vi "Create Sections and Channels.vi"(8 "error in (no error)":errorcluster, 10 "Configuration":T1={"Name"="", "Description"="", "Diagnostics Basic Configuraiton"={"Database File"=path "", "CAN Interface"=enum."CAN0", "Baud Rate"=0, "Diagnostic Protocol"=enum."GMLAN", "Transport Protocol"=enum."ISO TP - Normal Mode", "Transmit ID"=0, "Receive ID"=0, "Transmit Extension"=0, "Receive Extension"=0, "Receive UUDT ID"=0, "Enable Stream"=TRUE, "VW TP Channel ID"=0}, "DIDs"={"Description"="", "DIDPID Array"=[]}, "Input PIDs"={"Description"="", "DIDPID Array"=[]}, "Output PIDs"={"Description"="", "DIDPID Array"=[]}, "DPIDs"={"Description"="", "DPIDs"=[]}, "DTC"={"Description"="", "DTC descriptor"={"DTC Byte Length"=2, "Status Byte Length"=1, "Add Data Byte Length"=1, "Byte Order"=enum."Motorola"}}, "NI 986x Support"={"Enable 986x"=FALSE, "RIO Device"=0, "Bitfile"=path ""}, "Commands"={"Description"=""}, "Status"={"Description"=""}} {"Diagnostics Basic Configuraiton"."VW TP Channel ID" format="%.0x"; "Diagnostics Basic Configuraiton"."Receive UUDT ID" format="%.0x"; "Diagnostics Basic Configuraiton"."Receive Extension" format="%.0x"; "Diagnostics Basic Configuraiton"."Transmit Extension" format="%.0x"; "Diagnostics Basic Configuraiton"."Receive ID" format="%.0x"; "Diagnostics Basic Configuraiton"."Transmit ID" format="%.0x"; "DIDs"."DIDPID Array"."Signals"."Byte Order" items=["Little Endian", "Big Endian"]; "DIDs"."DIDPID Array"."Signals"."Data Type" items=["Signed", "Unsigned", "IEEE Float"]; "Input PIDs"."DIDPID Array"."Signals"."Byte Order" items=["Little Endian", "Big Endian"]; "Input PIDs"."DIDPID Array"."Signals"."Data Type" items=["Signed", "Unsigned", "IEEE Float"]; "Output PIDs"."DIDPID Array"."Signals"."Byte Order" items=["Little Endian", "Big Endian"]; "Output PIDs"."DIDPID Array"."Signals"."Data Type" items=["Signed", "Unsigned", "IEEE Float"]}, 11 "Device Item Ref in":T18 format="%.0x") -> (0 "error out":errorcluster, 3 "Device Item Ref out":T18 format="%.0x")   [LabVIEW 2013, in "Diagnostics Addon Shared.lvlib"]
uses:
  Diagnostics Addon Shared.lvlib
  <vilib>/NI Veristand/Custom Device API/Custom Device Item Ref.ctl
  Exported Configuration.ctl
  CAN Configuration.ctl
  CAN Interface.ctl
  Diagnostic Protocols.ctl
  Transport Protocols.ctl
  Exported DIDPIDs Cluster.ctl
  DIDPID Parameters.ctl
  DIDPID Signal Parameters.ctl
  Exported DPIDs Cluster.ctl
  Exported DPID Parameters.ctl
  DPID Parameters.ctl
  DPID Periodic Rate.ctl
  Exported DTC Cluster.ctl
  <vilib>/Automotive Diagnostic Command Set/Diagnostic Protocols.llb/DTC Descriptor.ctl
  Exported 986x Support.ctl
  Exported Command Cluster.ctl
  Exported Status Cluster.ctl
  <vilib>/NI Veristand/Custom Device API/Custom Device Channel.ctl
  <vilib>/NI Veristand/Custom Device API/Custom Device Channel Type.ctl
  FG Action.ctl
  GUID Lookup.vi
  <vilib>/NI Veristand/Custom Device API/NI VeriStand - Set Item Property.vi
  <vilib>/NI Veristand/Custom Device API/Set Item Property (Variant).vi
  <vilib>/NI Veristand/Custom Device API/Custom Device API.lvlib
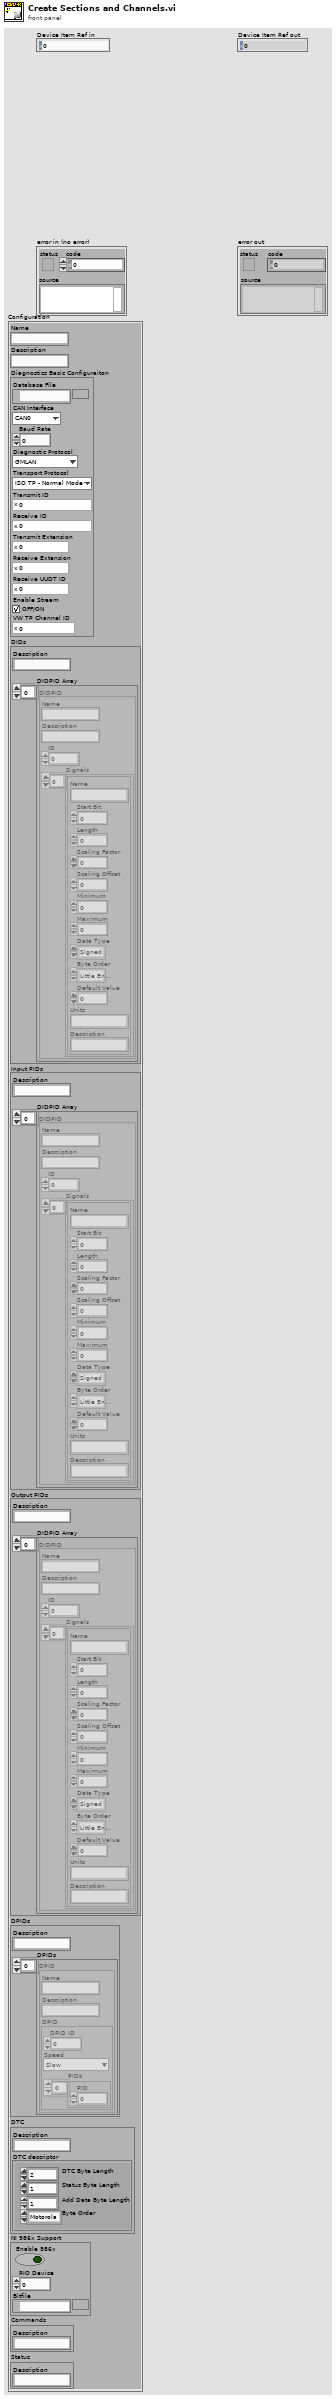
[diagram p1: front panel]
types:
  T1 = typedef "Diagnostics Addon Shared.lvlib/Exported Configuration.ctl" = cluster{"Name":string, "Description":string, "Diagnostics Basic Configuraiton":T2, "DIDs":T6, "Input PIDs":T6, "Output PIDs":T6, "DPIDs":T9, "DTC":T13, "NI 986x Support":T15, "Commands":T16, "Status":T17}
  T2 = typedef "Diagnostics Addon Shared.lvlib/CAN Configuration.ctl" = cluster{"Database File":path, "CAN Interface":T3, "Baud Rate":u32, "Diagnostic Protocol":T4, "Transport Protocol":T5, "Transmit ID":u32, "Receive ID":u32, "Transmit Extension":u8, "Receive Extension":u8, "Receive UUDT ID":u32, "Enable Stream":bool, "VW TP Channel ID":u32}
  T3 = typedef "Diagnostics Addon Shared.lvlib/CAN Interface.ctl" = enum16{"CAN0", "CAN1", "CAN2", "CAN3", "CAN4", "CAN5", "CAN6", "CAN7", "CAN8", "CAN9", "CAN10", "CAN11", "CAN12", "CAN13", "CAN14", "CAN15", "CAN16", "CAN17", "CAN18", "CAN19", "CAN20", "CAN21", "CAN22", "CAN23", "CAN24", "CAN25", "CAN26", "CAN27", "CAN28", "CAN29", "CAN30", "CAN31", "CAN32", "CAN33", "CAN34", "CAN35", "CAN36", "CAN37", "CAN38", "CAN39", "CAN40", "CAN41", "CAN42", "CAN43", "CAN44", "CAN45", "CAN46", "CAN47", "CAN48", "CAN49", "CAN50", "CAN51", "CAN52", "CAN53", "CAN54", "CAN55", "CAN56", "CAN57", "CAN58", "CAN59", "CAN60", "CAN61", "CAN62", "CAN63", "CAN 256 (Virtual)", "CAN 257 (Virtual)"}
  T4 = typedef "Diagnostics Addon Shared.lvlib/Diagnostic Protocols.ctl" = enum16{"GMLAN", "KWP-2000", "UDS"}
  T5 = typedef "Diagnostics Addon Shared.lvlib/Transport Protocols.ctl" = enum16{"ISO TP - Normal Mode", "ISO TP - Mixed Mode", "VW TP 2.0", "Diagnostics on IP"}
  T6 = typedef "Diagnostics Addon Shared.lvlib/Exported DIDPIDs Cluster.ctl" = cluster{"Description":string, "DIDPID Array":T7[]}
  T7 = typedef "Diagnostics Addon Shared.lvlib/DIDPID Parameters.ctl" = cluster{"Name":string, "Description":string, "ID":u16, "Signals":T8[]}
  T8 = typedef "Diagnostics Addon Shared.lvlib/DIDPID Signal Parameters.ctl" = cluster{"Name":string, "Start Bit":u8, "Length":u8, "Scaling Factor":dbl, "Scaling Offset":dbl, "Minimum":dbl, "Maximum":dbl, "Data Type":u32, "Byte Order":u32, "Default Value":dbl, "Units":string, "Description":string}
  T9 = typedef "Diagnostics Addon Shared.lvlib/Exported DPIDs Cluster.ctl" = cluster{"Description":string, "DPIDs":T10[]}
  T10 = typedef "Diagnostics Addon Shared.lvlib/Exported DPID Parameters.ctl" = cluster{"Name":string, "Description":string, "DPID":T11}
  T11 = typedef "Diagnostics Addon Shared.lvlib/DPID Parameters.ctl" = cluster{"DPID ID":u8, "Speed":T12, "PIDs":u16[]}
  T12 = typedef "Diagnostics Addon Shared.lvlib/DPID Periodic Rate.ctl" = enum16{"Slow", "Medium", "Fast"}
  T13 = typedef "Diagnostics Addon Shared.lvlib/Exported DTC Cluster.ctl" = cluster{"Description":string, "DTC descriptor":T14}
  T14 = typedef "DTC Descriptor.ctl" = cluster{"DTC Byte Length":i32, "Status Byte Length":i32, "Add Data Byte Length":i32, "Byte Order":enum16{"Motorola", "Intel"}}
  T15 = typedef "Diagnostics Addon Shared.lvlib/Exported 986x Support.ctl" = cluster{"Enable 986x":bool, "RIO Device":u16, "Bitfile":path}
  T16 = typedef "Diagnostics Addon Shared.lvlib/Exported Command Cluster.ctl" = cluster{"Description":string}
  T17 = typedef "Diagnostics Addon Shared.lvlib/Exported Status Cluster.ctl" = cluster{"Description":string}
  T18 = typedef "Custom Device API.lvlib/Custom Device Item Ref.ctl" = u64
  T19 = typedef "Diagnostics Addon Shared.lvlib/FG Action.ctl" = enum16{"Get", "Set"}
  T20 = typedef "Custom Device API.lvlib/Custom Device Channel.ctl" = cluster{"Type":T21, "Units":string, "Default Value":dbl, "Faultable":bool, "Scalable":bool}
  T21 = typedef "Custom Device API.lvlib/Custom Device Channel Type.ctl" = enum16{"Input", "Output"}
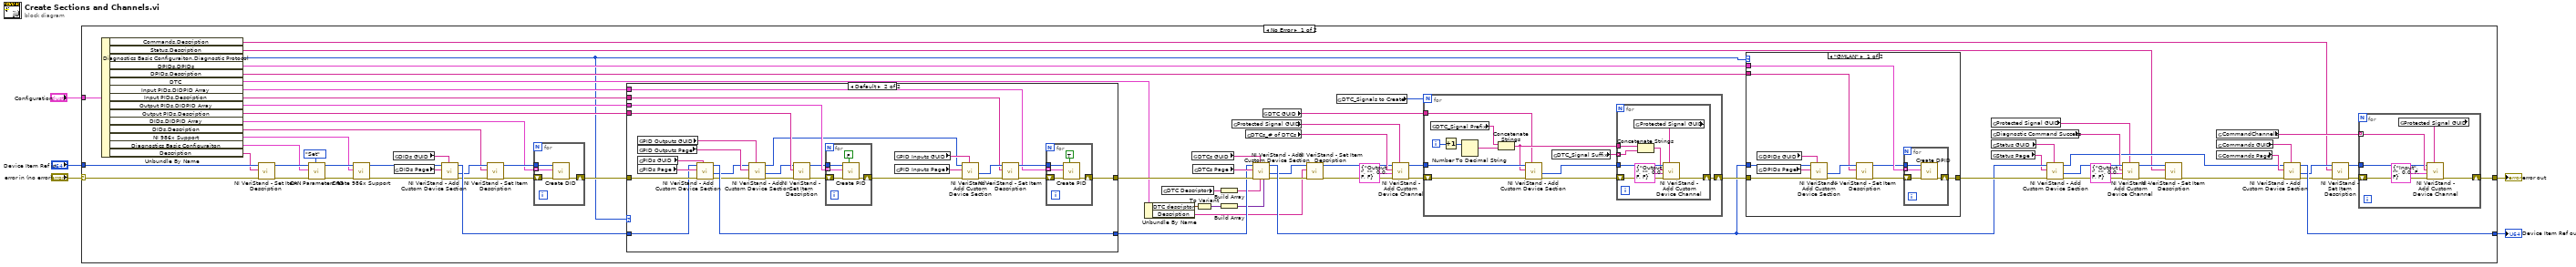
[diagram p0: block diagram]
diagram:
  n1 = case shown="No Error" "error in (no error)" {
    selector: "error in (no error)" -> [w44 w168]
    tunnel: [w54 w168] -> w4
    tunnel: "Device Item Ref in" -> [w48 w167]
    tunnel: [w52 w167] -> w2
    tunnel: "Configuration" -> [w47 _]
    frame No Error {
      n2 = Unbundle By Name(w47) -> ("Commands.Description"=w12:string, "Status.Description"=w13:string, "Diagnostics Basic Configuraiton.Diagnostic Protocol"=w6:T4, "DPIDs.DPIDs"=w22:T10[], "DPIDs.Description"=w21:string, "DTC"=w29:T13, "Input PIDs.DIDPID Array"=w32:T7[], "Input PIDs.Description"=w33:string, "Output PIDs.DIDPID Array"=w31:T7[], "Output PIDs.Description"=w34:string, "DIDs.DIDPID Array"=w35:T7[], "DIDs.Description"=w36:string, "NI 986x Support"=w7:T15, "Diagnostics Basic Configuraiton"=w42:T2, "Description"=w43:string)
      n3 = call <vilib>:"NI VeriStand - Set Item Description.vi"("error in (no error)"=w44, "Description"=w43, "Item Ref in"=w48) -> ("error out"=w45:errorcluster, "Item Ref out"=w46:T18)  [unwired: 6 in, 1 out]
      n4 = call "CAN Parameters FG.vi"("Action"=FG_Action."Set", "error in (no error)"=w45, "Diagnostics Basic Configuraiton"=w42, "Device Item Ref in"=w46) -> ("error out"=w11:errorcluster, "Device Item Ref out"=w8:T18)  [unwired: 5 in, 1 out]
      n5 = call "Create 986x Support.vi"("error in (no error)"=w11, "986x Support"=w7, "Device Item Ref in"=w8) -> ("error out"=w10:errorcluster, "Device Ref out"=w9:T18)  [unwired: 7 in]
      n6 = global read "GUID Lookup.vi" "DIDs GUID"() -> (w59:string)
      n7 = global read "GUID Lookup.vi" "DIDs Page"() -> (w60:string)
      n8 = call <vilib>:"NI VeriStand - Add Custom Device Section.vi"("GUID (Default Section)"=w59, "error in (no error)"=w10, "Section Name"=w60, "Parent Ref in"=w9) -> ("error out"=w40:errorcluster, "Section Ptr"=w38:T18, "Parent Ref out"=w57:T18)  [unwired: 4 in, 1 out]
      n9 = call <vilib>:"NI VeriStand - Set Item Description.vi"("error in (no error)"=w40, "Description"=w36, "Item Ref in"=w38) -> ("error out"=w39:errorcluster, "Item Ref out"=w37:T18)  [unwired: 6 in, 1 out]
      n10 = for {
        tunnel: w37 -> [w128]
        shift-right: [w129] -> w58
        shift-left: w39 -> [w130]
        tunnel: w35 -> [w127] mode=indexing
        n11 = call "Create DID.vi"("error in (no error)"=w130, "DIDPID"=w127, "Section Ptr"=w128) -> ("error out"=w129:errorcluster)  [unwired: 7 in, 1 out]
      }
      n12 = case shown="Default" w6 {
        tunnel: [w84 w106] -> w80
        tunnel: [w83 w105] -> w79
        tunnel: w58 -> [w84 w104]
        tunnel: w57 -> [w83 w103]
        tunnel: w34 -> [_ w97]
        tunnel: w33 -> [_ w92]
        tunnel: w32 -> [_ w91]
        tunnel: w31 -> [_ w90]
        frame "UDS" {
        }
        frame Default {
          n13 = global read "GUID Lookup.vi" "PID Outputs GUID"() -> (w102:string)
          n14 = global read "GUID Lookup.vi" "PID Outputs Page"() -> (w101:string)
          n15 = global read "GUID Lookup.vi" "PIDs GUID"() -> (w110:string)
          n16 = global read "GUID Lookup.vi" "PIDs Page"() -> (w109:string)
          n17 = call <vilib>:"NI VeriStand - Add Custom Device Section.vi"("GUID (Default Section)"=w110, "error in (no error)"=w104, "Section Name"=w109, "Parent Ref in"=w103) -> ("error out"=w100:errorcluster, "Section Ptr"=w99:T18, "Parent Ref out"=w105:T18)  [unwired: 4 in, 1 out]
          n18 = call <vilib>:"NI VeriStand - Add Custom Device Section.vi"("GUID (Default Section)"=w102, "error in (no error)"=w100, "Section Name"=w101, "Parent Ref in"=w99) -> ("error out"=w98:errorcluster, "Section Ptr"=w89:T18, "Parent Ref out"=w85:T18)  [unwired: 4 in, 1 out]
          n19 = call <vilib>:"NI VeriStand - Set Item Description.vi"("error in (no error)"=w98, "Description"=w97, "Item Ref in"=w89) -> ("error out"=w87:errorcluster, "Item Ref out"=w88:T18)  [unwired: 6 in, 1 out]
          n20 = for {
            tunnel: w88 -> [w113]
            shift-right: [w114] -> w86
            shift-left: w87 -> [w115]
            tunnel: w90 -> [w112] mode=indexing
            n21 = call "Create PID.vi"("Input?"=FALSE, "error in (no error)"=w115, "DIDPID"=w112, "Section Ptr"=w113) -> ("error out"=w114:errorcluster)  [unwired: 6 in, 1 out]
          }
          n22 = global read "GUID Lookup.vi" "PID Inputs GUID"() -> (w108:string)
          n23 = global read "GUID Lookup.vi" "PID Inputs Page"() -> (w107:string)
          n24 = call <vilib>:"NI VeriStand - Add Custom Device Section.vi"("GUID (Default Section)"=w108, "error in (no error)"=w86, "Section Name"=w107, "Parent Ref in"=w85) -> ("error out"=w96:errorcluster, "Section Ptr"=w94:T18)  [unwired: 4 in, 2 out]
          n25 = call <vilib>:"NI VeriStand - Set Item Description.vi"("error in (no error)"=w96, "Description"=w92, "Item Ref in"=w94) -> ("error out"=w95:errorcluster, "Item Ref out"=w93:T18)  [unwired: 6 in, 1 out]
          n26 = for {
            tunnel: w93 -> [w118]
            shift-right: [w119] -> w106
            shift-left: w95 -> [w120]
            tunnel: w91 -> [w117] mode=indexing
            n27 = call "Create PID.vi"("Input?"=TRUE, "error in (no error)"=w120, "DIDPID"=w117, "Section Ptr"=w118) -> ("error out"=w119:errorcluster)  [unwired: 6 in, 1 out]
          }
        }
      }
      n28 = Unbundle By Name(w29) -> ("DTC descriptor"=w28:T14, "Description"=w23:string)
      n29 = global read "GUID Lookup.vi" "DTC Descriptor"() -> (w30:string)
      n30 = global read "GUID Lookup.vi" "DTCs GUID"() -> (w81:string)
      n31 = global read "GUID Lookup.vi" "DTCs Page"() -> (w82:string)
      n32 = To Variant(anything=w28) -> (Variant=w78:variant)
      n33 = Build Array(w30) -> (w76:string[])
      n34 = Build Array(w78) -> (w77:variant[])
      n35 = global read "GUID Lookup.vi" "Protected Signal GUID"() -> (w50:string)
      n36 = global read "GUID Lookup.vi" "DTCs_# of DTCs"() -> (w74:string)
      n37 = call <vilib>:"NI VeriStand - Add Custom Device Section.vi"("Property Values"=w77, "Property names"=w76, "GUID (Default Section)"=w81, "error in (no error)"=w80, "Section Name"=w82, "Parent Ref in"=w79) -> ("error out"=w27:errorcluster, "Section Ptr"=w25:T18, "Parent Ref out"=w71:T18)  [unwired: 2 in, 1 out]
      n38 = global read "GUID Lookup.vi" "DTC GUID"() -> (w63:string)
      n39 = call <vilib>:"NI VeriStand - Set Item Description.vi"("error in (no error)"=w27, "Description"=w23, "Item Ref in"=w25) -> ("error out"=w26:errorcluster, "Item Ref out"=w24:T18)  [unwired: 6 in, 1 out]
      n40 = global read "GUID Lookup.vi" "DTC_Signals to Create"() -> (w61:i32)
      n41 = call <vilib>:"NI VeriStand - Add Custom Device Channel.vi"("GUID (Default Channel)"=w50, "error in (no error)"=w26, "Channel"=T20 {"Type"=enum."Output", "Units"="", "Default Value"=0.0, "Faultable"=FALSE, "Scalable"=FALSE}, "Channel Name"=w74, "Parent Ref in"=w24) -> ("error out"=w64:errorcluster, "Parent Ref out"=w62:T18)  [unwired: 3 in, 2 out]
      n42 = for {
        N: w61 -> [_]
        tunnel: w62 -> [w154]
        shift-right: [w158] -> w73
        shift-left: w64 -> [w152]
        tunnel: w63 -> [w149]
        i -> [w157]
        n43 = global read "GUID Lookup.vi" "DTC_Signal Prefix"() -> (w147:string)
        n44 = Increment(x=w157) -> (x+1=w156:i32)
        n45 = Number To Decimal String(number=w156) -> (decimal integer string=w155:string)  [unwired: 1 in]
        n46 = Concatenate Strings(w147, w155) -> (w150:string)
        n47 = call <vilib>:"NI VeriStand - Add Custom Device Section.vi"("GUID (Default Section)"=w149, "error in (no error)"=w152, "Section Name"=w150, "Parent Ref in"=w154) -> ("error out"=w151:errorcluster, "Section Ptr"=w153:T18)  [unwired: 4 in, 2 out]
        n48 = global read "GUID Lookup.vi" "DTC_Signal Suffix"() -> (w148:string[])
        n49 = for {
          tunnel: w153 -> [w164]
          tunnel: w150 -> [w161]
          tunnel: w148 -> [w162] mode=indexing
          shift-right: [w166] -> w158
          shift-left: w151 -> [w163]
          n50 = global read "GUID Lookup.vi" "Protected Signal GUID"() -> (w159:string)
          n51 = Concatenate Strings(w161, w162) -> (w160:string)
          n52 = call <vilib>:"NI VeriStand - Add Custom Device Channel.vi"("GUID (Default Channel)"=w159, "error in (no error)"=w163, "Channel"=T20 {"Type"=enum."Output", "Units"="", "Default Value"=0.0, "Faultable"=FALSE, "Scalable"=FALSE}, "Channel Name"=w160, "Parent Ref in"=w164) -> ("error out"=w166:errorcluster)  [unwired: 3 in, 3 out]
        }
      }
      n53 = case shown="\"GMLAN\"" w6 {
        tunnel: [w137 w146] -> w72
        tunnel: w73 -> [w139 w146]
        tunnel: w71 -> [w138 _]
        tunnel: w22 -> [w136 _]
        tunnel: w21 -> [w131 _]
        frame "GMLAN" {
          n54 = global read "GUID Lookup.vi" "DPIDs GUID"() -> (w141:string)
          n55 = global read "GUID Lookup.vi" "DPIDs Page"() -> (w140:string)
          n56 = call <vilib>:"NI VeriStand - Add Custom Device Section.vi"("GUID (Default Section)"=w141, "error in (no error)"=w139, "Section Name"=w140, "Parent Ref in"=w138) -> ("error out"=w135:errorcluster, "Section Ptr"=w133:T18)  [unwired: 4 in, 2 out]
          n57 = call <vilib>:"NI VeriStand - Set Item Description.vi"("error in (no error)"=w135, "Description"=w131, "Item Ref in"=w133) -> ("error out"=w134:errorcluster, "Item Ref out"=w132:T18)  [unwired: 6 in, 1 out]
          n58 = for {
            tunnel: w132 -> [w143]
            shift-right: [w144] -> w137
            shift-left: w134 -> [w145]
            tunnel: w136 -> [w142] mode=indexing
            n59 = call "Create DPID.vi"("error in (no error)"=w145, "DPID"=w142, "Section Ptr"=w143) -> ("error out"=w144:errorcluster)  [unwired: 7 in, 1 out]
          }
        }
        frame Default {
        }
      }
      n60 = global read "GUID Lookup.vi" "Protected Signal GUID"() -> (w49:string)
      n61 = global read "GUID Lookup.vi" "Diagnostic Command Success"() -> (w65:string)
      n62 = global read "GUID Lookup.vi" "Status GUID"() -> (w70:string)
      n63 = global read "GUID Lookup.vi" "Status Page"() -> (w69:string)
      n64 = call <vilib>:"NI VeriStand - Add Custom Device Section.vi"("GUID (Default Section)"=w70, "error in (no error)"=w72, "Section Name"=w69, "Parent Ref in"=w71) -> ("error out"=w66:errorcluster, "Section Ptr"=w67:T18, "Parent Ref out"=w53:T18)  [unwired: 4 in, 1 out]
      n65 = call <vilib>:"NI VeriStand - Add Custom Device Channel.vi"("GUID (Default Channel)"=w49, "error in (no error)"=w66, "Channel"=T20 {"Type"=enum."Output", "Units"="", "Default Value"=0.0, "Faultable"=FALSE, "Scalable"=FALSE}, "Channel Name"=w65, "Parent Ref in"=w67) -> ("error out"=w19:errorcluster, "Parent Ref out"=w20:T18)  [unwired: 3 in, 2 out]
      n66 = call <vilib>:"NI VeriStand - Set Item Description.vi"("error in (no error)"=w19, "Description"=w13, "Item Ref in"=w20) -> ("error out"=w18:errorcluster)  [unwired: 6 in, 2 out]
      n67 = global read "GUID Lookup.vi" "CommandChannels"() -> (w51:string[])
      n68 = global read "GUID Lookup.vi" "Commands GUID"() -> (w55:string)
      n69 = global read "GUID Lookup.vi" "Commands Page"() -> (w56:string)
      n70 = call <vilib>:"NI VeriStand - Add Custom Device Section.vi"("GUID (Default Section)"=w55, "error in (no error)"=w18, "Section Name"=w56, "Parent Ref in"=w53) -> ("error out"=w17:errorcluster, "Section Ptr"=w15:T18, "Parent Ref out"=w52:T18)  [unwired: 4 in, 1 out]
      n71 = call <vilib>:"NI VeriStand - Set Item Description.vi"("error in (no error)"=w17, "Description"=w12, "Item Ref in"=w15) -> ("error out"=w16:errorcluster, "Item Ref out"=w14:T18)  [unwired: 6 in, 1 out]
      n72 = for {
        tunnel: w51 -> [w126] mode=indexing
        tunnel: w14 -> [w124]
        shift-right: [w122] -> w54
        shift-left: w16 -> [w125]
        n73 = global read "GUID Lookup.vi" "Protected Signal GUID"() -> (w121:string)
        n74 = call <vilib>:"NI VeriStand - Add Custom Device Channel.vi"("GUID (Default Channel)"=w121, "error in (no error)"=w125, "Channel"=T20 {"Type"=enum."Input", "Units"="", "Default Value"=0.0, "Faultable"=FALSE, "Scalable"=FALSE}, "Channel Name"=w126, "Parent Ref in"=w124) -> ("error out"=w122:errorcluster)  [unwired: 3 in, 3 out]
      }
    }
    frame Error {
    }
  }
  "error out" <- w4
  "Device Item Ref out" <- w2
